vi "programa 5 archivoslvm.vi"() -> ()   [LabVIEW 2011]
panel:
  out "Array 2":dbl[](array[numeric])
  in  "lectura":bool
  in  "salir":bool
  in  "escribir":bool
  in  "rellenar":bool
  out "Array":dbl[](array[numeric])
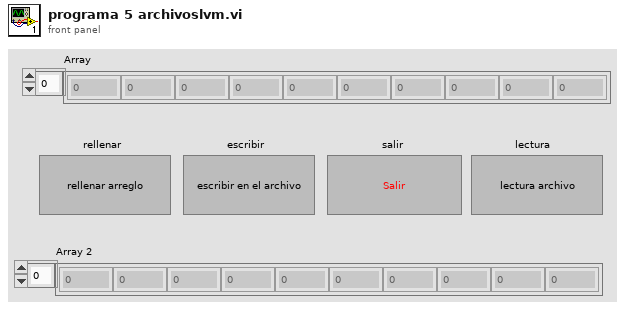
[diagram p1: front panel]
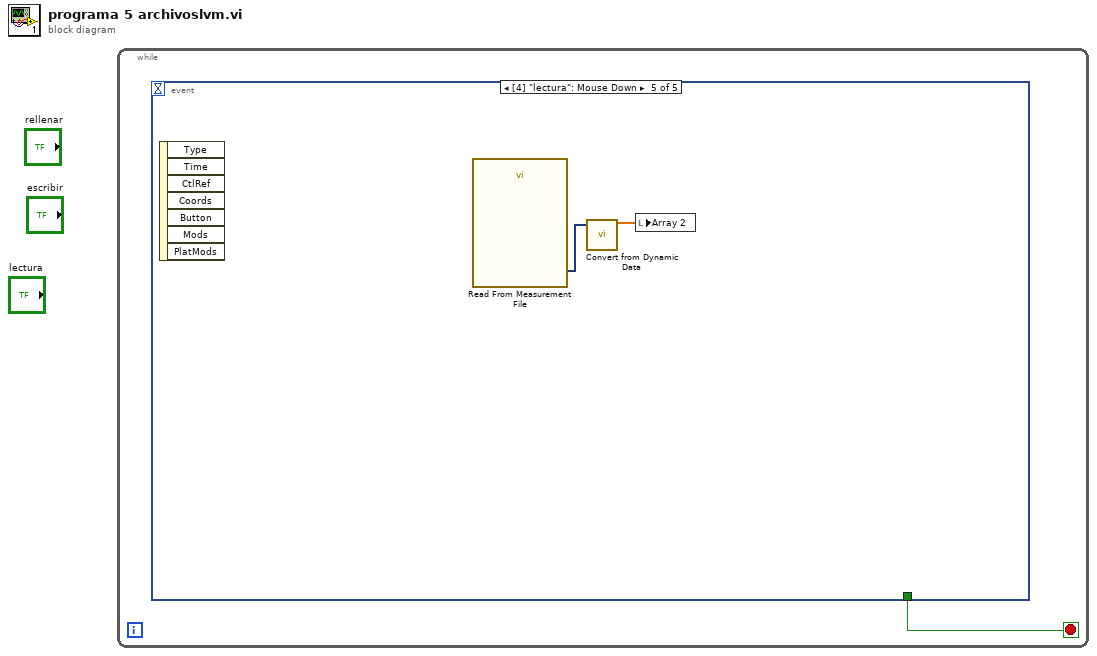
[diagram p0: block diagram]
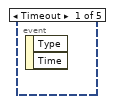
[diagram p2: hidden frame]
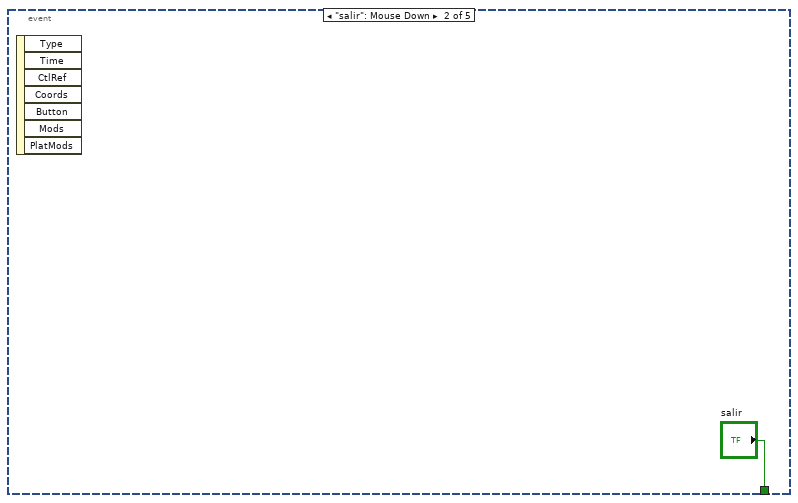
[diagram p3: hidden frame]
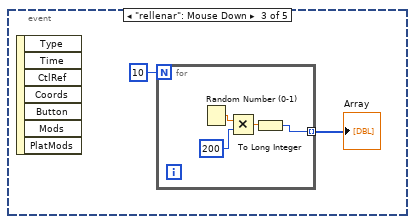
[diagram p4: hidden frame]
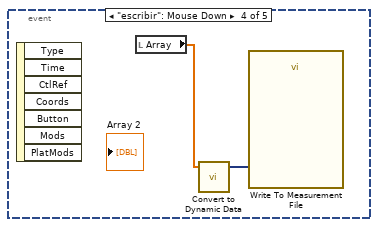
[diagram p5: hidden frame]
diagram:
  n1 = while {
    stop <- w1 stop-if-true
    n2 = event shown="[4] \"lectura\": Mouse Down" {
      selector: _ -> [_ _ _ _ _]
      dyn-events: _ -> [_ _ _ _ _]
      timeout: _ -> [_ _ _ _ _]
      tunnel: [_ "salir" _ _ _] -> w1
      event Timeout {
        n3 = event-data() -> ()  [unwired: 1 in, 2 out]
      }
      event "salir": Mouse Down {
        n4 = event-data() -> ()  [unwired: 1 in, 7 out]
      }
      event "rellenar": Mouse Down {
        n5 = event-data() -> ()  [unwired: 1 in, 7 out]
        n6 = for {
          N: 10 -> [_]
          tunnel: [w5] -> w3 mode=indexing
          n7 = Random Number (0-1)() -> (number: 0 to 1=w8:dbl)
          n8 = Multiply(x=w8, y=200) -> (x*y=w6:dbl)
          n9 = To Long Integer(number=w6) -> (32bit integer=w5:i32)
        }
        "Array" <- w3
      }
      event "escribir": Mouse Down {
        n10 = event-data() -> ()  [unwired: 1 in, 7 out]
        n11 = local read "Array"() -> (w10:dbl[])
        n12 = call "Convert to Dynamic Data"("Array"=w10) -> ("Dynamic Data Type"=w9:dynamicdata)  [unwired: 3 in]
        n13 = call "Write To Measurement File"("Signals"=w9) -> ()  [unwired: 16 in, 3 out]
      }
      event "lectura": Mouse Down {
        n14 = event-data() -> ()  [unwired: 1 in, 7 out]
        n15 = call "Read From Measurement File"() -> ("Signals"=w12:dynamicdata)  [unwired: 6 in, 5 out]
        n16 = call "Convert from Dynamic Data"("Dynamic Data Type"=w12) -> ("Array"=w11:dbl[])  [unwired: 3 in]
        n17 = local write "Array 2"(w11) -> ()
      }
    }
  }
